vi "Begin.vi"(8 "error in":errorcluster) -> (0 "error out":errorcluster)   [LabVIEW 2016]
doc: "Called before other user functions, this VI is expected to open initial I/O refnums, load in file data, and do all program initialization. Notice that the <B>error out</B> terminal is simply used for data flow. Wiring it to other structures or subVIs ensures that this VI runs first."
uses:
  <vilib>/Rock Robotics/WPI/Solenoid/WPI_SolenoidChannel.ctl
  <vilib>/Rock Robotics/SystemInterfaces/DIO/FPGA_DIOPWMChannel.ctl
  <vilib>/Rock Robotics/WPI/SafetyOutput/WPI_SafetyOutputConfigMenu.ctl
  <vilib>/Rock Robotics/WPI/DriverStation/WPI_DriverStationRobotMode2.ctl
  <vilib>/Rock Robotics/WPI/Joystick/WPI_JoystickDeviceEnum.ctl
  <vilib>/Rock Robotics/SystemInterfaces/DIO/FPGA_DIOChannel.ctl
  <vilib>/Rock Robotics/SystemInterfaces/spilib/spi_bus.ctl
  <vilib>/Rock Robotics/SystemInterfaces/AI/FPGA_AIChannel.ctl
  Google Drive/HowdyBots-Share/BotStuff/2017_SteamWorks/Code/BotCode/Active/Robot Global Data.vi
  <vilib>/Rock Robotics/Network Tables/NT Write String Array.vi
  <vilib>/Rock Robotics/WPI/RobotDrive/WPI_RobotDriveOpen4MotorWithVictorSP.vi
  <vilib>/Rock Robotics/WPI/Solenoid/WPI_SolenoidOpenSingle.vi
  <vilib>/Rock Robotics/WPI/MotorControl/WPI_MotorControlOpen SPARK.vi
  <vilib>/Rock Robotics/Network Tables/NT Write Number.vi
  <vilib>/Rock Robotics/WPI/Switch/WPI_SwitchOpenLimit.vi
  <vilib>/Rock Robotics/WPI/Counter/WPI_CounterDigitalInputToDigitalSource.vi
  PDP Currents Variable.vi
  <vilib>/Rock Robotics/WPI/Gyro/WPI_GyroXRS450_SPI_Open.vi
  <vilib>/Rock Robotics/WPI/Ultrasonic/WPI_SonarMB1010AnalogOpen.vi
  <vilib>/Rock Robotics/WPI/Ultrasonic/WPI_SonarMB1010AnalogRefNum Registry Set.vi
  <vilib>/Rock Robotics/WPI/Utilities/WPI_GetSetVariantRefNum.vi
  <vilib>/Rock Robotics/WPI/Gyro/WPI_GyroAnalogOpen.vi
  <vilib>/Rock Robotics/SystemInterfaces/AI/FPGA_AIGyroChannel.ctl
panel:
  in  "Solenoid Channel 4":T1=enum."Solenoid 3"
  in  "Solenoid Channel 3":T1=enum."Solenoid 2"
  in  "Solenoid Channel 2":T1=enum."Solenoid 1"
  in  "Solenoid Channel":T1
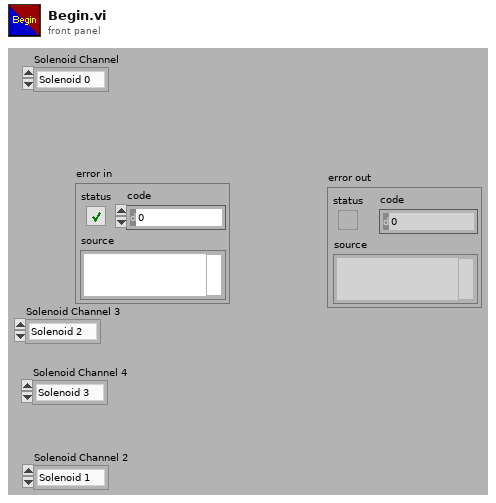
[diagram p1: front panel]
types:
  T1 = typedef "WPI_SolenoidChannel.ctl" = enum8{"Solenoid 0", "Solenoid 1", "Solenoid 2", "Solenoid 3", "Solenoid 4", "Solenoid 5", "Solenoid 6", "Solenoid 7", "Invalid"}
  T2 = typedef "FPGA_DIOChannel.ctl" = enum8{"DIO 0", "DIO 1", "DIO 2", "DIO 3", "DIO 4", "DIO 5", "DIO 6", "DIO 7", "DIO 8", "DIO 9", "DIO MXP 0", "DIO MXP 1", "DIO MXP 2", "DIO MXP 3", "DIO MXP 4", "DIO MXP 5", "DIO MXP 6", "DIO MXP 7", "DIO MXP 8", "DIO MXP 9", "DIO MXP 10", "DIO MXP 11", "DIO MXP 12", "DIO MXP 13", "DIO MXP 14", "DIO MXP 15", "SPI Port CS1", "SPI Port CS2", "SPI Port CS3", "SPI Port MISO", "SPI Port MOSI", "Invalid"}
  T3 = typedef "FPGA_AIChannel.ctl" = enum8{"AI 0", "AI 1", "AI 2", "AI 3", "AI MXP 0", "AI MXP 1", "AI MXP 2", "AI MXP 3", "Invalid"}
  T4 = typedef "spi_bus.ctl" = enum16{"SPI On-Board, CS0", "SPI On-Board, CS1", "SPI On-Board, CS2", "SPI On-Board, CS3", "SPI MXP", "Invalid"}
  T5 = typedef "WPI_SafetyOutputConfigMenu.ctl" = enum16{"Enable", "Disable"}
  T6 = typedef "FPGA_DIOPWMChannel.ctl" = enum8{"PWM 0", "PWM 1", "PWM 2", "PWM 3", "PWM 4", "PWM 5", "PWM 6", "PWM 7", "PWM 8", "PWM 9", "PWM MXP 0", "PWM MXP 1", "PWM MXP 2", "PWM MXP 3", "PWM MXP 4", "PWM MXP 5", "PWM MXP 6", "PWM MXP 7", "PWM MXP 8", "PWM MXP 9", "Invalid"}
  T7 = typedef "WPI_JoystickDeviceEnum.ctl" = enum16{"USB 0", "USB 1", "USB 2", "USB 3", "USB 4", "USB 5"}
  T8 = typedef "WPI_DriverStationRobotMode2.ctl" = enum16{"Autonomous Disabled", "Autonomous Enabled", "Teleop Disabled", "Teleop Enabled", "Disconnected", "Finish", "Test Disabled", "Test Enabled", "Emergency Stopped"}
  T9 = typedef "WPI_CompressorDevRef.ctl" = cluster{"DevStatus":errorcluster, "Pneumatics Control Module":u8}
  T10 = typedef "WPI_JoystickDevRef.ctl" = cluster{"Device":T7}
  T11 = typedef "WPI_MotorControlDeviceRef.ctl" = cluster{"DeviceStatus":errorcluster, "Type":T12, "PWM":cluster{"PWM Channel":T6, "DeadBand":T13}, "CAN":cluster{"Device Number":u8, "SetOutput VI Ref":variant, "GetOutput VI Ref":variant, "Enable VI Ref":variant, "Disable VI Ref":variant, "Data":variant}, "Invert":bool}
  T12 = typedef "WPI_MotorControlType.ctl" = enum16{"PWM", "CAN"}
  T13 = typedef "WPI_PWMDeadband.ctl" = cluster{"Name":string, "maxPositivePwm":i32, "minPositivePwm":i32, "centerPwm":i32, "maxNegativePwm":i32, "minNegativePwm":i32, "angularRange":u16}
  T14 = typedef "WPI_SolenoidDevRef.ctl" = cluster{"DevStatus":errorcluster, "Pneumatics Control Module":u8, "Forward Solenoid Channel":T1, "Reverse Solenoid Channel":T1}
  T15 = typedef "WPI_RobotDriveDevRef.ctl" = cluster{"DevStatus":errorcluster, "Motors[]":T11[], "Square Inputs":bool, "Max Output":dbl}
  T16 = typedef "WPI_SonarMB1010AnalogDeviceRef.ctl" = cluster{"AIDeviceRef":T17, "Scaling factor (V/in)":dbl, "Average Bits":u8}
  T17 = typedef "WPI_AnalogChannelDevRef.ctl" = cluster{"DevStatus":errorcluster, "Analog Channel":T3}
  T18 = typedef "WPI_DigitalInputDevRef.ctl" = cluster{"DevStatus":errorcluster, "DIO Channel":T2}
  T19 = typedef "FPGA_CounterEncoderSourceConvertionLVSourceType.ctl" = cluster{"DevStatus":errorcluster, "AnalogTriggerMode?":bool, "DigitalMode":cluster{"DIO Channel":T20}, "AnalogTriggerMode":cluster{"AnalogTriggerIndex":T21, "OutputType":T22}}
  T20 = typedef "FPGA_DIODigitalSourceChannel.ctl" = enum8{"DIO 0", "DIO 1", "DIO 2", "DIO 3", "DIO 4", "DIO 5", "DIO 6", "DIO 7", "DIO 8", "DIO 9", "DIO MXP 0", "DIO MXP 1", "DIO MXP 2", "DIO MXP 3", "DIO MXP 4", "DIO MXP 5", "DIO MXP 6", "DIO MXP 7", "DIO MXP 8", "DIO MXP 9", "DIO MXP 10", "DIO MXP 11", "DIO MXP 12", "DIO MXP 13", "DIO MXP 14", "DIO MXP 15", "Disabled"}
  T21 = typedef "FPGA_AnalogTriggerIndex.ctl" = enum8{"Trig 0", "Trig 1", "Trig 2", "Trig 3", "Trig 4", "Trig 5", "Trig 6", "Trig 7", "Invalid"}
  T22 = typedef "FPGA_AnalogTriggerOutType.ctl" = enum16{"InWindow", "TriggerState", "Rising", "Falling"}
  T23 = typedef "FPGA_AIGyroChannel.ctl" = enum8{"AI 0", "AI 1", "Invalid"}
  T24 = typedef "WPI_GyroDevRef.ctl" = cluster{"DevStatus":errorcluster, "Analog Channel":T3, "Offset":dbl, "Gain (VoltsPerDegree/Second)":dbl, "Gyro Type":enum16{"Analog", "XRS450"}, "Handle":i32, "SPI Bus":T4, "Device Found":bool, "Sample Rate":dbl, "Calibrate On Open":bool}
  T25 = typedef "WPI_SwitchDevRef.ctl" = cluster{"DevStatus":errorcluster, "DIO Channel":T2, "CntIndex":T26, "Normally Closed":bool}
  T26 = typedef "FPGA_CounterCtrSystemIndex.ctl" = enum8{"Ctr 0", "Ctr 1", "Ctr 2", "Ctr 3", "Ctr 4", "Ctr 5", "Ctr 6", "Ctr 7", "Invalid"}
  T27 = typedef "WPI_EncoderDevRef.ctl" = cluster{"DevStatus":errorcluster, "EncoderIndex":T28, "CounterIndex":T26, "DistancePerCount":dbl, "Decoding Type":T29}
  T28 = typedef "FPGA_EncoderIdx.ctl" = enum8{"Enc 0", "Enc 1", "Enc 2", "Enc 3", "Enc 4", "Enc 5", "Enc 6", "Enc 7", "Invalid"}
  T29 = typedef "WPI_EncoderType.ctl" = enum16{"1x", "2x", "4x"}
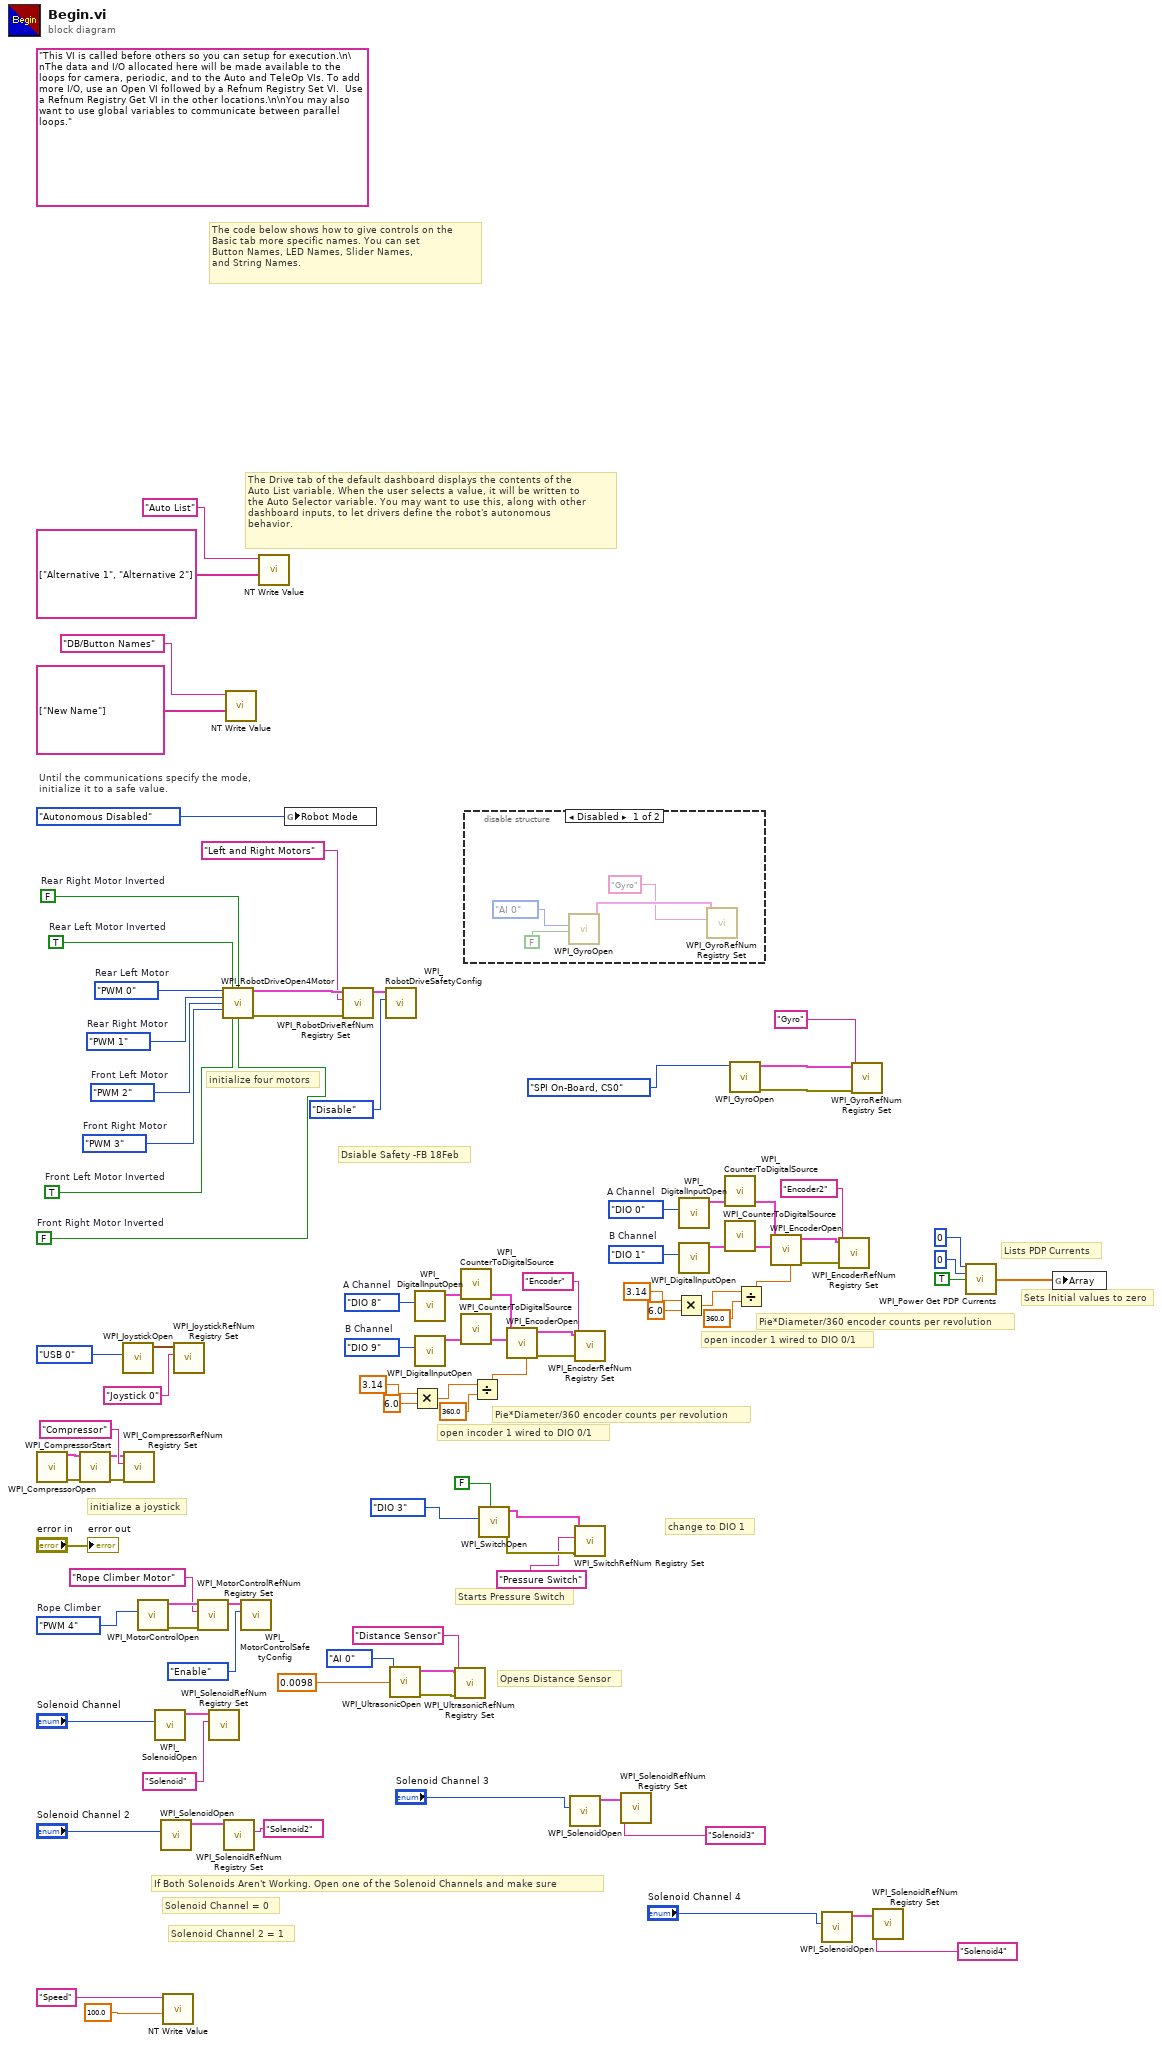
[diagram p0: block diagram]
diagram:
  w20 = FPGA_DIOChannel."DIO 1"  # B Channel
  w19 = FPGA_DIOChannel."DIO 0"  # A Channel
  w47 = FPGA_DIOChannel."DIO 9"  # B Channel
  w46 = FPGA_DIOChannel."DIO 8"  # A Channel
  w63 = FPGA_DIOPWMChannel."PWM 4"  # Rope Climber
  w72 = TRUE  # Front Left Motor Inverted
  w73 = FALSE  # Front Right Motor Inverted
  w74 = FPGA_DIOPWMChannel."PWM 3"  # Front Right Motor
  w77 = FPGA_DIOPWMChannel."PWM 2"  # Front Left Motor
  (unwired) "This VI is called before others so you can setup for execution.\n\nThe data and I/O allocated here will be made available to the loops for camera, periodic, and to the Auto and TeleOp VIs. To add more I/O, use an Open VI followed by a Refnum Registry Set VI.  Use a Refnum Registry Get VI in the other locations.\n\nYou may also want to use global variables to communicate between parallel loops."
  w89 = FPGA_DIOPWMChannel."PWM 1"  # Rear Right Motor
  w90 = FPGA_DIOPWMChannel."PWM 0"  # Rear Left Motor
  w93 = TRUE  # Rear Left Motor Inverted
  w75 = FALSE  # Rear Right Motor Inverted
  # "Pie*Diameter/360 encoder counts per revolution"
  # "open incoder 1 wired to DIO 0/1"
  # "Pie*Diameter/360 encoder counts per revolution"
  # "Dsiable Safety -FB 18Feb"
  # "Opens Distance Sensor"
  # "Sets Initial values to zero"
  # "Lists PDP Currents"
  # "open incoder 1 wired to DIO 0/1"
  # "change to DIO 1"
  # "Starts Pressure Switch"
  # "Solenoid Channel 2 = 1"
  # "Solenoid Channel = 0"
  # "If Both Solenoids Aren't Working. Open one of the Solenoid Channels and make sure"
  # "The Drive tab of the default dashboard displays the contents of the\nAuto List variable. When the user selects a value, it will be written to\nthe Auto Selector variable. You may want to use this, along with other\ndashboard inputs, to let drivers define the robot's autonomous\nbehavior."
  # "The code below shows how to give controls on the\nBasic tab more specific names. You can set\nButton Names, LED Names, Slider Names,\nand String Names."
  # "initialize a joystick"
  # "Until the communications specify the mode,\ninitialize it to a safe value."
  # "initialize four motors"
  n1 = call <vilib>:"WPI_CompressorOpen.vi"() -> ("CompressorDevRef"=w68:T9, "error out"=w67:errorcluster)  [unwired: 14 in]
  n2 = call <vilib>:"WPI_CompressorStart.vi"("error in (no error)"=w67, "CompressorDevRef"=w68) -> ("error out"=w69:errorcluster, "CompressorDevRef"=w70:T9)  [unwired: 8 in]
  n3 = call <vilib>:"WPI_JoystickOpen.vi"("JoystickDevice"=WPI_JoystickDeviceEnum."USB 0") -> ("JoystickDevRef"=w84:T10)  [unwired: 10 in]
  n4 = call <vilib>:"WPI_CompressorRefNum Registry Set.vi"("error in (no error)"=w69, "refnum name"="Compressor", "CompressorDevRef"=w70) -> ()  [unwired: 7 in, 2 out]
  n5 = call-poly <vilib>:"WPI_MotorControlOpen.vi"("PWM Channel"=w63) -> ("error out"=w59:errorcluster, "MotorControlDeviceRef"=w62:T11)  [unwired: 9 in]
  n6 = call-poly <vilib>:"WPI_SolenoidOpen.vi"("Solenoid Channel"="Solenoid Channel") -> ("SolenoidDevRef"=w65:T14)  [unwired: 9 in, 1 out]
  n7 = call-poly <vilib>:"WPI_SolenoidOpen.vi"("Solenoid Channel"="Solenoid Channel 2") -> ("SolenoidDevRef"=w57:T14)  [unwired: 9 in, 1 out]
  n8 = call-poly <vilib>:"NT Write Value.vi"("Numeric"=100.0, "Name"="Speed") -> ()  [unwired: 9 in, 1 out]
  n9 = call <vilib>:"WPI_JoystickRefNum Registry Set.vi"("refnum name"="Joystick 0", "JoystickDevRef"=w84) -> ()  [unwired: 8 in, 2 out]
  n10 = call <vilib>:"WPI_MotorControlRefNum Registry Set.vi"("error in (no error)"=w59, "refnum name"="Rope Climber Motor", "MotorControlDevRef"=w62) -> ("MotorControlDevRef"=w61:T11)  [unwired: 7 in, 1 out]
  n11 = call <vilib>:"WPI_SolenoidRefNum Registry Set.vi"("refnum name"="Solenoid", "SolenoidDevRef"=w65) -> ()  [unwired: 8 in, 2 out]
  n12 = call-poly <vilib>:"WPI_RobotDriveOpen4Motor.vi"("Rear Left Motor"=w90, "Rear Left Motor Inverted"=w93, "Rear Right Motor Inverted"=w75, "Rear Right Motor"=w89, "Front Left Motor"=w77, "Front Right Motor"=w74, "Front Left Motor Inverted"=w72, "Front Right Motor Inverted"=w73) -> ("RobotDriveDevRef"=w92:T15, "error out"=w76:errorcluster)  [unwired: 6 in]
  n13 = call <vilib>:"WPI_SolenoidRefNum Registry Set.vi"("refnum name"="Solenoid2", "SolenoidDevRef"=w57) -> ()  [unwired: 8 in, 2 out]
  n14 = call-poly <vilib>:"NT Write Value.vi"("String Array"=string[] ["New Name"], "Name"="DB/Button Names") -> ()  [unwired: 9 in, 1 out]
  n15 = call <vilib>:"WPI_MotorControlSafetyConfig.vi"("mode"=WPI_SafetyOutputConfigMenu."Enable", "MotorControlDevRef"=w61) -> ()  [unwired: 8 in, 2 out]
  n16 = call-poly <vilib>:"NT Write Value.vi"("String Array"=string[] ["Alternative 1", "Alternative 2"], "Name"="Auto List") -> ()  [unwired: 9 in, 1 out]
  n17 = global write "Robot Global Data.vi" "Robot Mode"(WPI_DriverStationRobotMode2."Autonomous Disabled" ("Robot Mode")) -> ()
  n18 = call <vilib>:"WPI_RobotDriveRefNum Registry Set.vi"("error in (no error)"=w76, "refnum name"="Left and Right Motors", "RobotDriveDevRef"=w92) -> ("RobotDriveDevRef"=w88:T15)  [unwired: 1 in, 7 out]
  n19 = call <vilib>:"WPI_RobotDriveSafetyConfig.vi"("mode"=WPI_SafetyOutputConfigMenu."Disable", "RobotDriveDevRef"=w88) -> ()  [unwired: 8 in, 2 out]
  n20 = call-poly <vilib>:"WPI_UltrasonicOpen.vi"("Scaling factor (V/in)"=0.0098, "Analog Channel"=FPGA_AIChannel."AI 0") -> ("error out"=w27:errorcluster, "SonarMB1010AnalogDevRef"=w30:T16)  [unwired: 8 in]
  n21 = Multiply(x=3.14, y=6.0) -> (x*y=w23:dbl)
  n22 = call <vilib>:"WPI_DigitalInputOpen.vi"("DIO Channel"=w46) -> ("DigitalInputDevRef"=w43:T18)  [unwired: 1 in, 9 out]
  n23 = call <vilib>:"WPI_DigitalInputOpen.vi"("DIO Channel"=w47) -> ("DigitalInputDevRef"=w44:T18)  [unwired: 1 in, 9 out]
  n24 = call-poly <vilib>:"WPI_UltrasonicRefNum Registry Set.vi"("error in (no error)"=w27, "refnum name"="Distance Sensor", "SonarMB1010AnalogDevRef"=w30) -> ()  [unwired: 7 in, 2 out]
  n25 = call-poly <vilib>:"WPI_CounterToDigitalSource.vi"("DigitalInputDevRef"=w43) -> ("Digital Source"=w42:T19)  [unwired: 6 out]
  n26 = call-poly <vilib>:"WPI_CounterToDigitalSource.vi"("DigitalInputDevRef"=w44) -> ("Digital Source"=w45:T19)  [unwired: 6 out]
  n27 = disable-structure shown="Disabled" {
    frame Disabled {
      n28 = call-poly <vilib>:"WPI_GyroOpen.vi"("Calibrate On Open"=FALSE, "Analog Channel"=FPGA_AIGyroChannel."AI 0") -> ("GyroDevRef"=w97:T24)  [unwired: 7 in, 2 out]
      n29 = call <vilib>:"WPI_GyroRefNum Registry Set.vi"("refnum name"="Gyro", "GyroDevRef"=w97) -> ()  [unwired: 8 in, 2 out]
    }
    frame Enabled {
    }
  }
  n30 = Divide(x=w23, y=360.0) -> (x/y=w21:dbl)
  n31 = call-poly <vilib>:"WPI_SwitchOpen.vi"("Normally Closed"=FALSE, "DIO Channel"=FPGA_DIOChannel."DIO 3") -> ("error out"=w49:errorcluster, "SwitchDevRef"=w50:T25)  [unwired: 8 in]
  n32 = call <vilib>:"WPI_EncoderOpen.vi"("DistancePerCount"=w21, "BSource"=w45, "ASource"=w42) -> ("error out"=w39:errorcluster, "EncoderDevRef"=w41:T27)  [unwired: 5 in, 2 out]
  n33 = call-poly <vilib>:"WPI_SolenoidOpen.vi"("Solenoid Channel"="Solenoid Channel 3") -> ("SolenoidDevRef"=w6:T14)  [unwired: 9 in, 1 out]
  n34 = call <vilib>:"WPI_EncoderRefNum Registry Set.vi"("error in (no error)"=w39, "refnum name"="Encoder", "EncoderDevRef"=w41) -> ()  [unwired: 7 in, 2 out]
  n35 = call <vilib>:"WPI_SwitchRefNum Registry Set.vi"("error in (no error)"=w49, "refnum name"="Pressure Switch", "SwitchDevRef"=w50) -> ()  [unwired: 7 in, 2 out]
  n36 = call <vilib>:"WPI_SolenoidRefNum Registry Set.vi"("refnum name"="Solenoid3", "SolenoidDevRef"=w6) -> ()  [unwired: 8 in, 2 out]
  n37 = Multiply(x=3.14, y=6.0) -> (x*y=w9:dbl)
  n38 = call <vilib>:"WPI_DigitalInputOpen.vi"("DIO Channel"=w19) -> ("DigitalInputDevRef"=w16:T18)  [unwired: 1 in, 9 out]
  n39 = call <vilib>:"WPI_DigitalInputOpen.vi"("DIO Channel"=w20) -> ("DigitalInputDevRef"=w17:T18)  [unwired: 1 in, 9 out]
  n40 = call-poly <vilib>:"WPI_CounterToDigitalSource.vi"("DigitalInputDevRef"=w16) -> ("Digital Source"=w15:T19)  [unwired: 6 out]
  n41 = call-poly <vilib>:"WPI_CounterToDigitalSource.vi"("DigitalInputDevRef"=w17) -> ("Digital Source"=w18:T19)  [unwired: 6 out]
  n42 = call-poly <vilib>:"WPI_GyroOpen.vi"("SPI Bus"=spi_bus."SPI On-Board, CS0") -> ("error out"=w34:errorcluster, "GyroDevRef"=w33:T24)  [unwired: 9 in]
  n43 = Divide(x=w9, y=360.0) -> (x/y=w7:dbl)
  n44 = call <vilib>:"WPI_EncoderOpen.vi"("DistancePerCount"=w7, "BSource"=w18, "ASource"=w15) -> ("error out"=w12:errorcluster, "EncoderDevRef"=w14:T27)  [unwired: 5 in, 2 out]
  n45 = call-poly <vilib>:"WPI_SolenoidOpen.vi"("Solenoid Channel"="Solenoid Channel 4") -> ("SolenoidDevRef"=w3:T14)  [unwired: 9 in, 1 out]
  n46 = call <vilib>:"WPI_EncoderRefNum Registry Set.vi"("error in (no error)"=w12, "refnum name"="Encoder2", "EncoderDevRef"=w14) -> ()  [unwired: 7 in, 2 out]
  n47 = call <vilib>:"WPI_GyroRefNum Registry Set.vi"("error in (no error)"=w34, "refnum name"="Gyro", "GyroDevRef"=w33) -> ()  [unwired: 7 in, 2 out]
  n48 = call <vilib>:"WPI_SolenoidRefNum Registry Set.vi"("refnum name"="Solenoid4", "SolenoidDevRef"=w3) -> ()  [unwired: 8 in, 2 out]
  n49 = call <vilib>:"WPI_Power Get PDP Currents.vi"("Power Distribution Panel (0)"=u8 0, "PDP Channel"=0, "Tare Currents?"=TRUE) -> ("all currents (A)"=w35:dbl[])  [unwired: 10 in, 2 out]
  n50 = global write "PDP Currents Variable.vi" "Array"(w35) -> ()
  "error out" <- "error in"
